vi "errorClusterContent.vi"() -> ()   [LabVIEW 2014]
panel:
  out "status":bool
  out "source":string
  out "code":i32
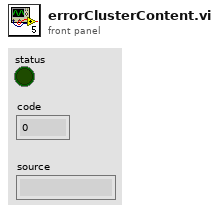
[diagram p1: front panel]
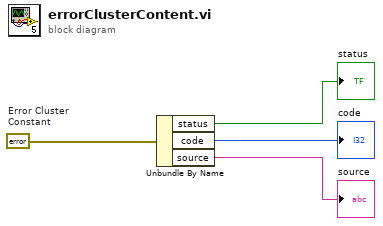
[diagram p0: block diagram]
diagram:
  w4 = errorcluster {"status"=FALSE, "code"=0, "source"=""}  # Error Cluster Constant
  n1 = Unbundle By Name "Unbundle By Name"(w4) -> ("status"=→"status":bool, "code"=→"code":i32, "source"=→"source":string)
